vi "Main_FGV_All Data.vi"(7 "Data_Action":T5, 8 "Error in":errorcluster, 11 "All Data In":cluster{"User Account Data":T1}={"User Account Data"={"帳號 :"="", "權限等級："=enum."開發人員", "建立時間："="", "修改時間："="", "到期時間："="", "狀態："=enum."可使用", "期限："=enum."一天", "密碼："=""}}) -> (0 "Error Out":errorcluster, 3 "All Data Out":cluster{"User Account Data":T1}={"User Account Data"={"帳號 :"="", "權限等級："=enum."開發人員", "建立時間："="", "修改時間："="", "到期時間："="", "狀態："=enum."可使用", "期限："=enum."一天", "密碼："=""}})   [LabVIEW 2015]
uses:
  0.Main_Control/Control_Main_All Data.ctl
  2.User Accounts/Control_User account_Data.ctl
  2.User Accounts/Control_User account_Permissions.ctl
  2.User Accounts/Control_User Accounts_Status.ctl
  2.User Accounts/Control_User account_Date.ctl
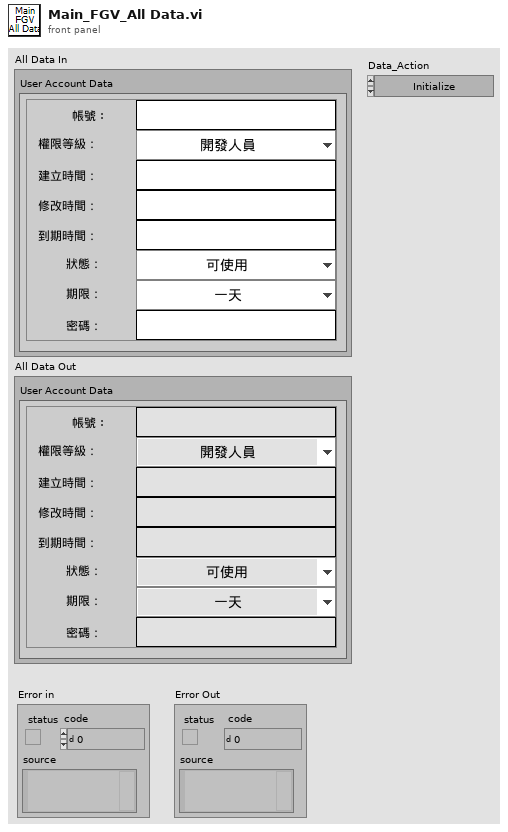
[diagram p1: front panel]
types:
  T1 = typedef "Control_User account_Data.ctl" = cluster{"帳號 :":string, "權限等級：":T2, "建立時間：":string, "修改時間：":string, "到期時間：":string, "狀態：":T3, "期限：":T4, "密碼：":string}
  T2 = typedef "Control_User account_Permissions.ctl" = enum16{"開發人員", "管理者", "工程師", "作業員"}
  T3 = typedef "Control_User Accounts_Status.ctl" = enum16{"可使用", "不可使用"}
  T4 = typedef "Control_User account_Date.ctl" = enum16{"零天", "一天", "七天", "一個月", "一年", "三年"}
  T5 = typedef "Control_Main_All Data.ctl" = enum16{"Initialize", "Set Data", "Get Data"}
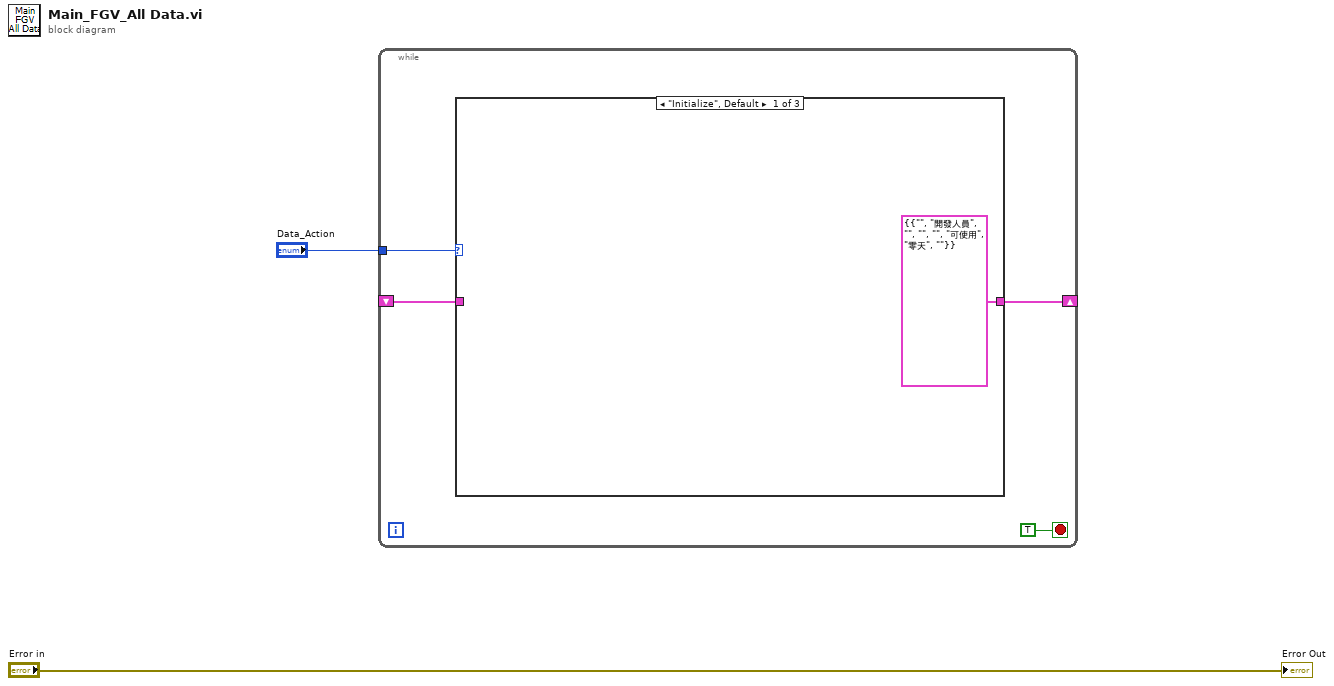
[diagram p0: block diagram]
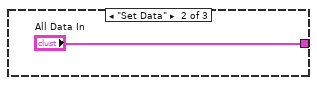
[diagram p2: hidden frame]
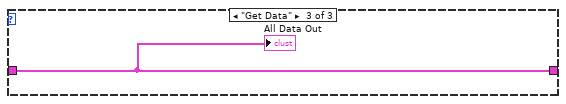
[diagram p3: hidden frame]
diagram:
  n1 = while {
    tunnel: "Data_Action" -> [w5]
    shift-right: [w4] -> _
    shift-left: _ -> [w3]
    stop <- TRUE stop-if-true
    n2 = case shown="\"Initialize\", Default" w5 {
      tunnel: [cluster{"User Account Data":T1} {"User Account Data"={"帳號 :"="", "權限等級："=enum."開發人員", "建立時間："="", "修改時間："="", "到期時間："="", "狀態："=enum."可使用", "期限："=enum."零天", "密碼："=""}} ("All Data In") "All Data In" w9] -> w4
      tunnel: w3 -> [_ _ w9]
      frame "Initialize", Default {
      }
      frame "Set Data" {
      }
      frame "Get Data" {
        "All Data Out" <- w9
      }
    }
  }
  "Error Out" <- "Error in"
